vi "uNotify Optimize.vi"(8 "error in (no error)":errorcluster, 10 "Listener Transport":refnum<class "uTransport.lvclass">, 11 "uNotifyMode in":refnum<class "uNotifyMode.lvclass">) -> (0 "error out":errorcluster, 3 "uNotifyMode out":refnum<class "uNotifyMode.lvclass">)   [LabVIEW 2021, in "uFramework.lvlib" / "uNotifyMode.lvclass"]
doc: "Call this VI to force the object to optimize its execution for the type of the listener transport; in order to improve the data throughput."
uses:
  uNotifyMode.lvclass
  uTransport/uTransport.lvclass
  uNotifyMode.lvclass/uNotifyMode.ctl
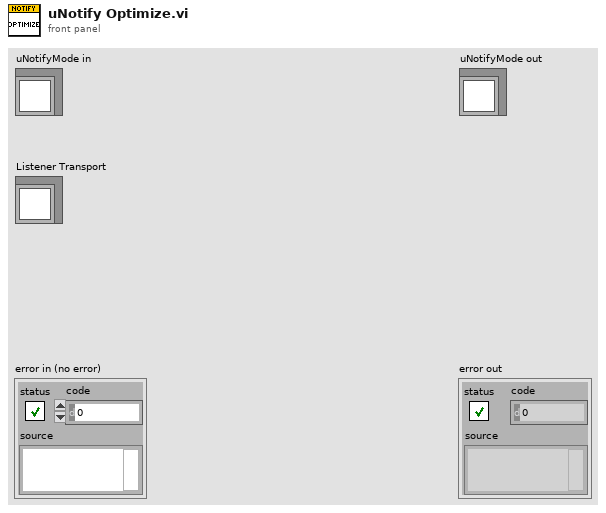
[diagram p1: front panel]
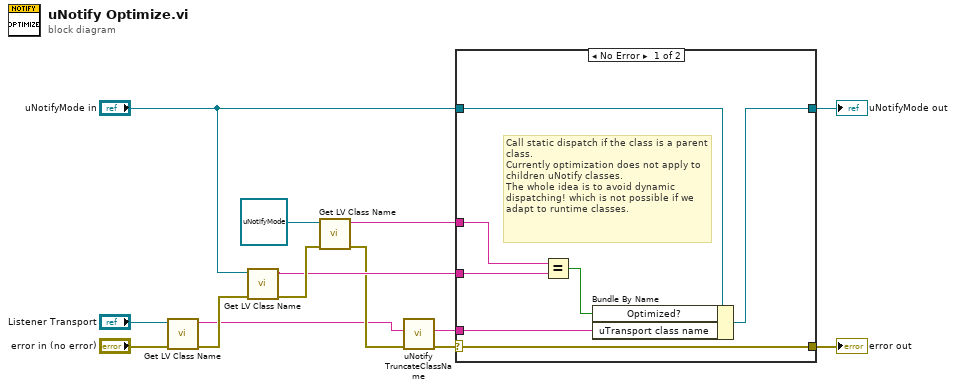
[diagram p0: block diagram]
diagram:
  n1 = call <vilib>:"Get LV Class Name.vi"("error in (no error)"="error in (no error)", "object"="Listener Transport") -> ("error out"=w9:errorcluster, "class name"=w2:string)  [unwired: 8 in]
  n2 = call <vilib>:"Get LV Class Name.vi"("error in (no error)"=w9, "object"="uNotifyMode in") -> ("error out"=w8:errorcluster, "class name"=w6:string)  [unwired: 8 in]
  n3 = call <vilib>:"Get LV Class Name.vi"("error in (no error)"=w8, "object"=refnum<class "uNotifyMode.lvclass"> refnum ("uBroker.lvlib:uNotifyMode.lvclass")) -> ("error out"=w4:errorcluster, "class name"=w5:string)  [unwired: 8 in]
  n4 = call "uNotify TruncateClassName.vi"("error in (no error)"=w4, "LV Class Name in"=w2) -> ("error out"=w3:errorcluster, "LV Class Name out"=w1:string)  [unwired: 8 in]
  n5 = case shown="No Error" w3 {
    selector: w3 -> [w21 w23]
    tunnel: [w21 w23] -> w14
    tunnel: [w19 w22] -> w13
    tunnel: "uNotifyMode in" -> [w18 w22]
    tunnel: w1 -> [w20 _]
    tunnel: w6 -> [w17 _]
    tunnel: w5 -> [w16 _]
    frame No Error {
      # "Call static dispatch if the class is a parent class.\nCurrently optimization does not apply to children uNotify classes.\nThe whole idea is to avoid dynamic dispatching! which is not possible if we adapt to runtime classes."
      n6 = Equal?(x=w16, y=w17) -> (x = y?=w15:bool)
      n7 = Bundle By Name(cluster=w18, "Optimized?"=w15, "uTransport class name"=w20) -> (w19:refnum<class "uNotifyMode.lvclass">)
    }
    frame Error {
    }
  }
  "error out" <- w14
  "uNotifyMode out" <- w13
